vi "ParseProjectString.vi"() -> ()   [LabVIEW 2017, in "BuildServer.lvlib" / "BuildServer.lvclass"]
uses:
  BuildServer.lvclass
panel:
  out "BuildSpec Name":string
  out "Target Name":string
  out "Project Name":string
  in  "ProjectString":string
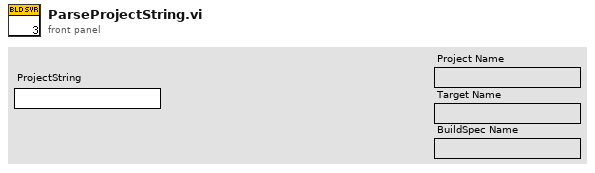
[diagram p1: front panel]
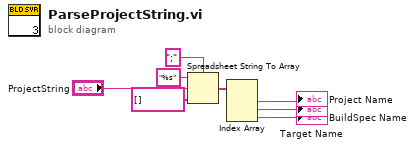
[diagram p0: block diagram]
diagram:
  n1 = Spreadsheet String To Array(delimiter (Tab)=";", format string="%s", spreadsheet string="ProjectString", array type (2D Dbl)=string[] []) -> (array=w6:string[])
  n2 = Index Array(array=w6) -> (element #1=→"Project Name":string, element #2=→"Target Name":string, element #3=→"BuildSpec Name":string)  [unwired: 3 in]
